vi "Choreo_TrajectoryDifferential_GetTrajSample.vi"(9 "index":i32, 11 "ChoreoTrajectoryDifferential":T2) -> (3 "ChoreoDifferentialSample":T1={"timestamp"=-999.0, "x"=0.0, "y"=0.0, "heading"=0.0, "velocityL"=0.0, "velocityR"=0.0, "angularVelocity"=0.0, "accelL"=0.0, "accelR"=0.0, "accelAngular"=0.0, "forceL"=0.0, "forceR"=0.0})   [LabVIEW 2019, in "ChoreoLib.lvlib"]
doc: "Return a particular Differential trajectory sample\n\nInputs:\n -- ChoreoTrajectoryDifferential - cluster - data cluster for this trajectory \n -- index - integer - zero relative index into the array of samples\n\nOutputs:\n -- ChoreoDifferentialSample - cluster - selected trajectory sample"
uses:
  ChoreoLib.lvlib
  TypeDef/ChoreoTrajectoryDifferential.ctl
  TypeDef/ChoreoDifferentialSample.ctl
  TypeDef/ChoreoEventMarker.ctl
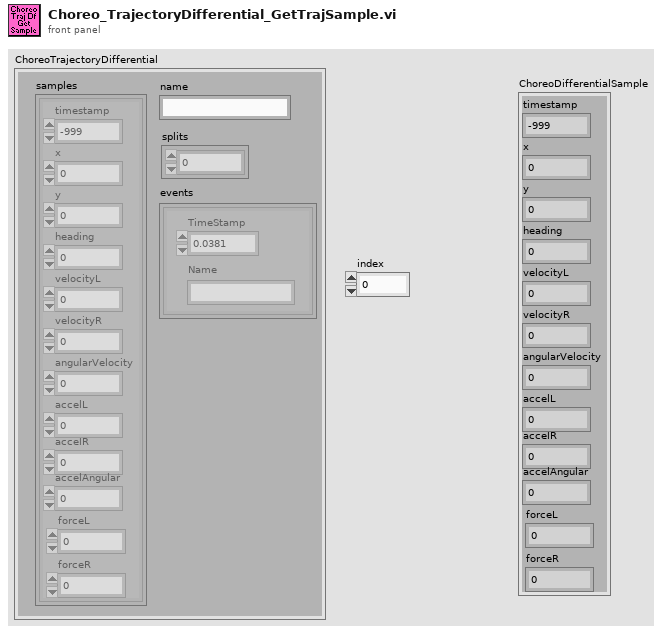
[diagram p1: front panel]
types:
  T1 = typedef "ChoreoLib.lvlib/ChoreoDifferentialSample.ctl" = cluster{"timestamp":dbl, "x":dbl, "y":dbl, "heading":dbl, "velocityL":dbl, "velocityR":dbl, "angularVelocity":dbl, "accelL":dbl, "accelR":dbl, "accelAngular":dbl, "forceL":dbl, "forceR":dbl}
  T2 = typedef "ChoreoLib.lvlib/ChoreoTrajectoryDifferential.ctl" = cluster{"name":string, "samples":T1[], "splits":i32[], "events":T3[]}
  T3 = typedef "ChoreoLib.lvlib/ChoreoEventMarker.ctl" = cluster{"TimeStamp":dbl, "Name":string}
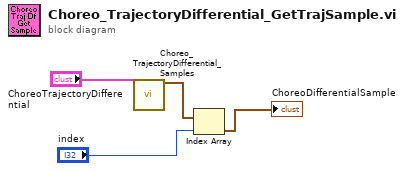
[diagram p0: block diagram]
diagram:
  n1 = call "Choreo_TrajectoryDifferential_Samples.vi"("ChoreoTrajectoryDifferential"="ChoreoTrajectoryDifferential") -> ("samples"=w2:T1[])  [unwired: 10 in]
  n2 = Index Array(array=w2, index="index") -> (element=→"ChoreoDifferentialSample":T1)
